vi "Areotech move abs.vi"(7 "speed":dbl, 8 "error in (no error)":errorcluster, 9 "stage index":i32, 10 "position":dbl, 11 "AerotechStage in":refnum<class "AerotechStage.lvclass">) -> (0 "error out":errorcluster, 3 "AerotechStage out":refnum<class "AerotechStage.lvclass">)   [LabVIEW 2020, in "AerotechStage.lvclass"]
uses:
  AerotechStage.lvclass
  AerotechStage.lvclass/AerotechStage.ctl
  EnableSingle.vi
  DisableSingle.vi
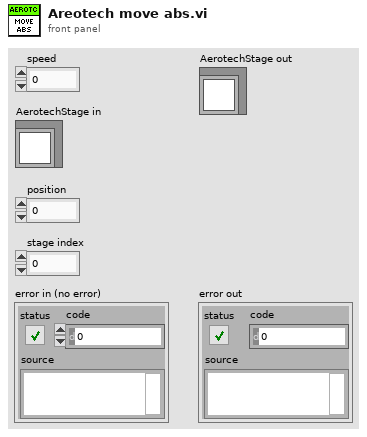
[diagram p1: front panel]
types:
  T1 = typedef "OnOffTypeDef.ctl" = enum16{"off", "on"}
  T2 = typedef "ControllerDiagPacket.ctl" = cluster{"Count":i32, "Packet Time":i64, "Axes":T3[], "error":errorcluster}
  T3 = typedef "AxisDiagPacket.ctl" = cluster{"Axis Name":string, "Acceleration Command":dbl, "Amplifier Temperature":sgl, "Analog Input 0":dbl, "Analog Input 1":dbl, "Analog Output 0":dbl, "Analog Output 1":dbl, "Axis Fault (num)":i32, "Axis Fault (str)":string, "Axis Fault (bits)":cluster{"AmplifierFault":bool, "AmplifierTemperatureFault":bool, "CcwEndOfTravelLimitFault":bool, "CcwSoftwareLimitFault":bool, "CommunicationLostFault":bool, "CwEndOfTravelLimitFault":bool, "CwSoftwareLimitFault":bool, "EmergencyStopFault":bool, "EncoderFault":bool, "ExternalFault":bool, "FeedbackScalingFault":bool, "HallSensorFault":bool, "MarkerSearchFault":bool, "MaxVelocityCommandFault":bool, "MotorTemperatureFault":bool, "None":bool, "OverCurrentFault":bool, "PositionErrorFault":bool, "PositionFeedbackFault":bool, "PowerSupplyFault":bool, "VelocityErrorFault":bool, "VelocityFeedbackFault":bool, "VoltageClampFault":bool}, "Axis Status (num)":i32, "Axis Status (str)":string, "Axis Status (bits)":cluster{"AccelerationPhase":bool, "AutofocusActive":bool, "BrakeOutput":bool, "CalibrationActive":bool, "CalibrationEnabled":bool, "CcwEndOfTravelLimitInput":bool, "CommandShapingFilterDone":bool, "CosineEncoderError":bool, "CurrentClamp":bool, "CwEndOfTravelLimitInput":bool, "DecelerationPhase":bool, "EmergencyStopInput":bool, "Enabled":bool, "GantryMasterActive":bool, "GantryModeActive":bool, "HallAInput":bool, "HallBInput":bool, "HallCInput":bool, "Homed":bool, "HomeLimitInput":bool, "Homing":bool, "InPosition":bool, "InPosition2":bool, "JoystickControl":bool, "MarkerInput":bool, "MasterMotionSuppressed":bool, "MasterSlaveControl":bool, "MotionIsCw":bool, "MoveActive":bool, "None":bool, "PositionCaptureActive":bool, "ServoControl":bool, "SineEncoderError":bool}, "Current Command":sgl, "Current Error":sgl, "Current Feedback":sgl, "Digital Input 0":i32, "Digital Input 1":i32, "Digital Input 2":i32, "Digital Output 0":i32, "Digital Output 1":i32, "Digital Output 2":i32, "Position Feedback Auxiliary":dbl, "Position Command":dbl, "Position Error":dbl, "Position Feedback":dbl, "Program Position Command":dbl, "Program Position Error":dbl, "Program Position Feedback":dbl, "Velocity Command":dbl, "Velocity Error":dbl, "Velocity Feedback":dbl}
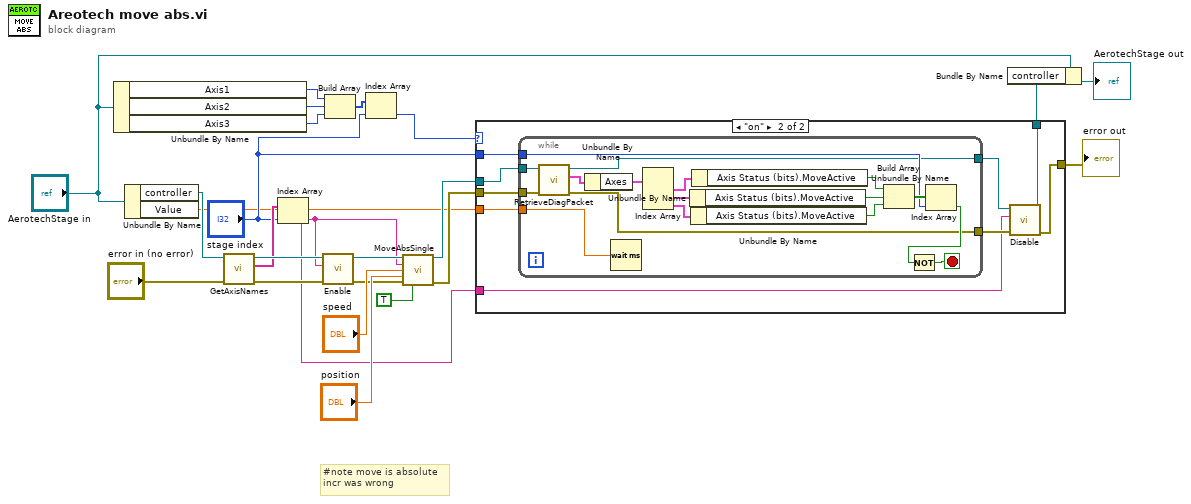
[diagram p0: block diagram]
diagram:
  # "#note move is absolute\nincr was wrong"
  n1 = Unbundle By Name("AerotechStage in") -> ("Axis1"=w14:T1, "Axis2"=w13:T1, "Axis3"=w12:T1)
  n2 = Unbundle By Name("AerotechStage in") -> ("controller"=w21:refnum<k24>, "Value"=w1:dbl)
  n3 = call "GetAxisNames.vi"("error in (no error)"="error in (no error)", "controller in"=w21) -> ("error out"=w17:errorcluster, "axis names"=w16:string[], "controller out"=w18:refnum<k24>)  [unwired: 7 in]
  n4 = Index Array(array=w16, index="stage index") -> (element=w8:string)
  n5 = call-poly "Enable.vi"("error in (no error)"=w17, "axis name"=w8, "controller in"=w18) -> ("error out"=w10:errorcluster, "controller out"=w19:refnum<k24>)  [unwired: 7 in]
  n6 = Build Array(w14, w13, w12) -> (w11:T1[])
  n7 = Index Array(array=w11, index="stage index") -> (element=w3:T1)
  n8 = call "MoveAbsSingle.vi"("controller in"=w19, "axis name"=w8, "speed"="speed", "distance"="position", "error in (no error)"=w10, "return immediately"=TRUE) -> ("controller out"=w6:refnum<k24>, "error out"=w5:errorcluster)  [unwired: 8 in]
  n9 = case shown="\"on\"" w3 {
    tunnel: [w26 w29] -> w7
    tunnel: [w25 w28] -> w9
    tunnel: w8 -> [_ w31]
    tunnel: w6 -> [w25 w35]
    tunnel: w5 -> [w26 w34]
    tunnel: "stage index" -> [_ w33]
    tunnel: w1 -> [_ w27]
    frame "off", Default {
    }
    frame "on" {
      n10 = while {
        tunnel: w35 -> [w43]
        tunnel: w34 -> [w42]
        tunnel: w33 -> [w41]
        tunnel: [w38] -> w32
        tunnel: [w37] -> w30
        tunnel: w27 -> [w36]
        stop <- w39 stop-if-true
        n11 = call "RetrieveDiagPacket.vi"("error in (no error)"=w42, "Controller In"=w43) -> ("error out"=w38:errorcluster, "ControllerDiagPacket"=w44:T2, "Controller Out"=w37:refnum<k24>)  [unwired: 7 in]
        n12 = Unbundle By Name(w44) -> ("Axes"=w45:T3[])
        n13 = Wait (ms)(milliseconds to wait=w36) -> ()  [unwired: 1 out]
        n14 = Index Array(array=w45) -> (element #1=w46:T3, element #2=w47:T3, element #3=w48:T3)  [unwired: 3 in]
        n15 = Unbundle By Name(w47) -> ("Axis Status (bits).MoveActive"=w50:bool)
        n16 = Unbundle By Name(w48) -> ("Axis Status (bits).MoveActive"=w51:bool)
        n17 = Unbundle By Name(w46) -> ("Axis Status (bits).MoveActive"=w49:bool)
        n18 = Build Array(w49, w50, w51) -> (w52:bool[])
        n19 = Index Array(array=w52, index=w41) -> (element=w40:bool)
        n20 = Not(x=w40) -> (.not. x?=w39:bool)
      }
      n21 = call-poly "Disable.vi"("error in (no error)"=w32, "axis name"=w31, "controller in"=w30) -> ("error out"=w29:errorcluster, "controller out"=w28:refnum<k24>)  [unwired: 7 in]
    }
  }
  "error out" <- w7
  n22 = Bundle By Name(cluster="AerotechStage in", "controller"=w9) -> (→"AerotechStage out":refnum<class "AerotechStage.lvclass">)
